vi "Timing-Get High Resolution Relative Time.vi"(11 "error in (no error)":errorcluster) -> (8 "double precision float":dbl, 15 "error out":errorcluster)   [LabVIEW 2020]
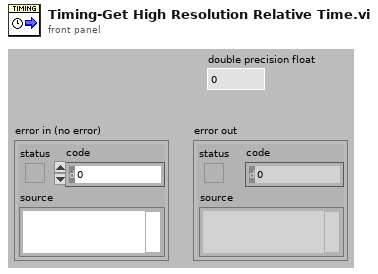
[diagram p1: front panel]
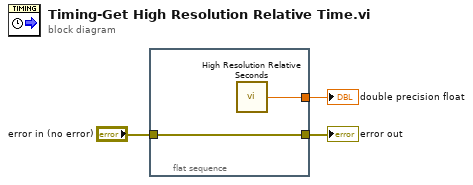
[diagram p0: block diagram]
diagram:
  n1 = flat-sequence {
    tunnel: [w4] -> w3
    tunnel: "error in (no error)" -> [w5]
    tunnel: [w5] -> w1
    frame #0 {
      n2 = call <vilib>:"High Resolution Relative Seconds.vi"() -> ("relative seconds"=w4:dbl)
    }
  }
  "error out" <- w1
  "double precision float" <- w3
